vi "song_processing.vi"() -> ()   [LabVIEW 2019]
panel:
  out "x-y":waveform(dbl)
  out "size(s) 2":i32
  out "size(s)":i32
  out "data":waveform(dbl)[](array[waveform])
  in  "path":path
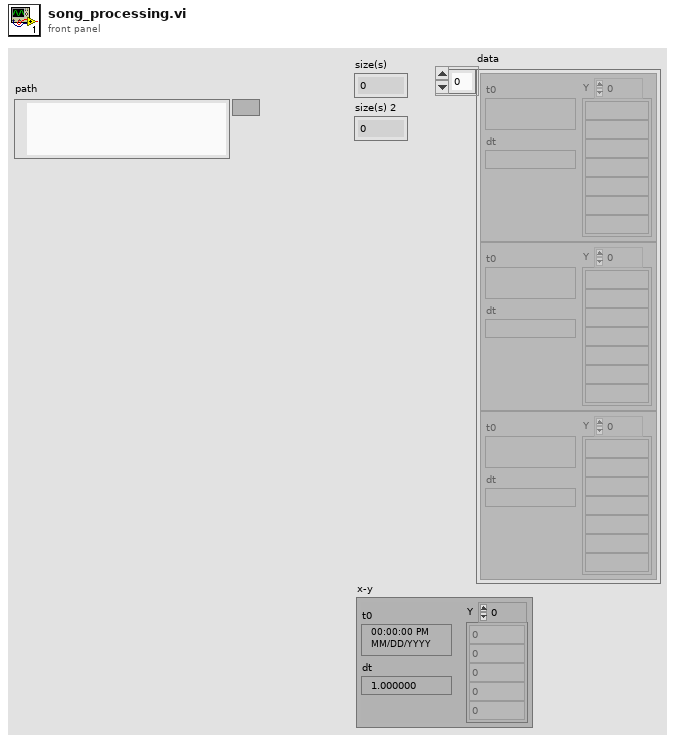
[diagram p1: front panel]
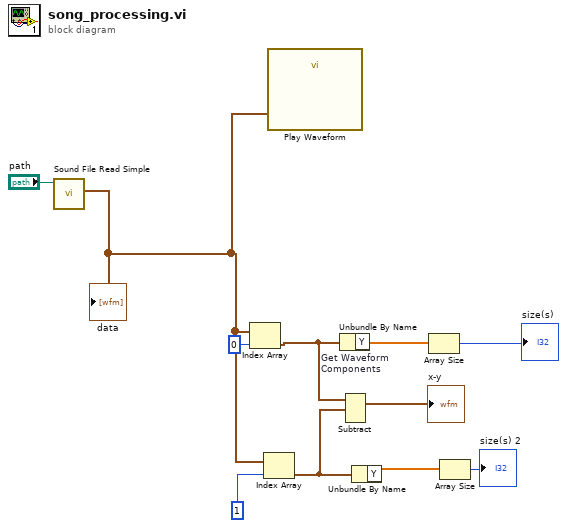
[diagram p0: block diagram]
diagram:
  n1 = call <vilib>:"Sound File Read Simple.vi"("path"="path") -> ("data"=w4:waveform(dbl)[])  [unwired: 7 in, 3 out]
  "data" <- w4
  n2 = Index Array(array=w4, index=0) -> (element=w3:waveform(dbl))
  n3 = Index Array(array=w4, index=1) -> (element=w2:waveform(dbl))
  n4 = call "Play Waveform"("Data"=w4) -> ()  [unwired: 18 in, 1 out]
  n5 = Unbundle By Name "Get Waveform Components"(w3) -> ("Y"=w8:dbl[])
  n6 = Subtract(1:w2, 2:w3) -> (0:→"x-y":waveform(dbl))  [unwired: 1 in, 1 out]
  n7 = Unbundle By Name(w2) -> ("Y"=w7:dbl[])
  n8 = Array Size(array=w8) -> (size(s)=→"size(s)":i32)
  n9 = Array Size(array=w7) -> (size(s)=→"size(s) 2":i32)
